vi "Auto Check Each Tube.vi"(0 "Ch 0 Leak":dbl, 1 "Cur Ch 0":refnum<vi>, 2 "Cur Ch 1":refnum<vi>, 5 "Tube #":i32, 7 "Ch 1 Leak":dbl, 9 "Barcodes in":string[](array[string]), 11 "BoardHandle in":T1, 12 "error in (no error)":errorcluster) -> (3 "Bool Bad Tubes":bool[](array[boolean]), 6 "Bad Tubes":string[](array[string]), 10 "error out":errorcluster, 13 "Channel 1 current":dbl, 14 "Channel 0 current":dbl, 15 "BoardHandle out":T1)   [LabVIEW 2020]
uses:
  Program Files/National Instruments/LabVIEW 2018/instr.lib/CAEN PSM/CAEN PSM.lvlib
panel:
  in  "User":string
  # "OUTPUTS"
  # "INPUTS"
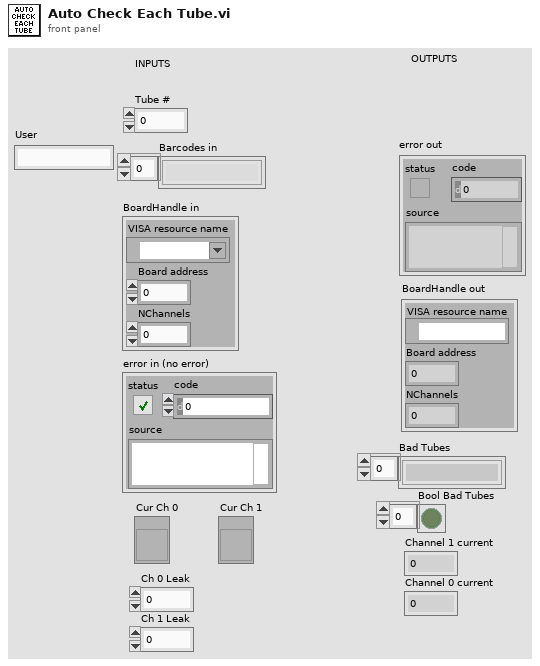
[diagram p1: front panel]
types:
  T1 = cluster{"VISA resource name":refnum<visa-resource-name>, "Board address":u8, "NChannels":u8}
  T2 = typedef "CAEN PSM.lvlib/BoardHandle.ctl" = cluster{"VISA resource name":refnum<visa-resource-name>, "Board address":u8, "NChannels":u8}
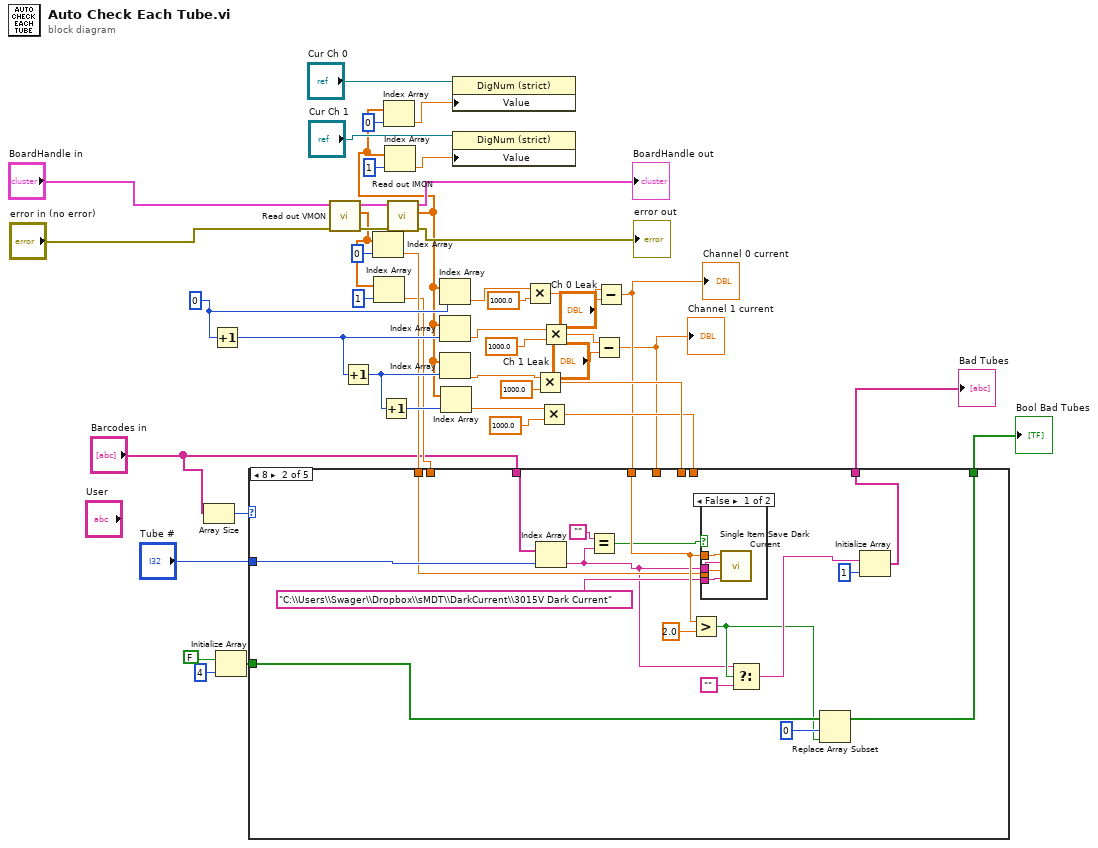
[diagram p0: block diagram]
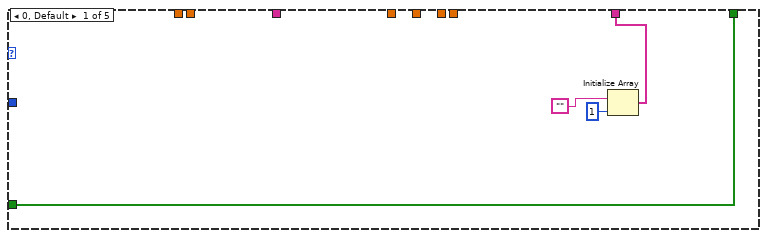
[diagram p2: hidden frame]
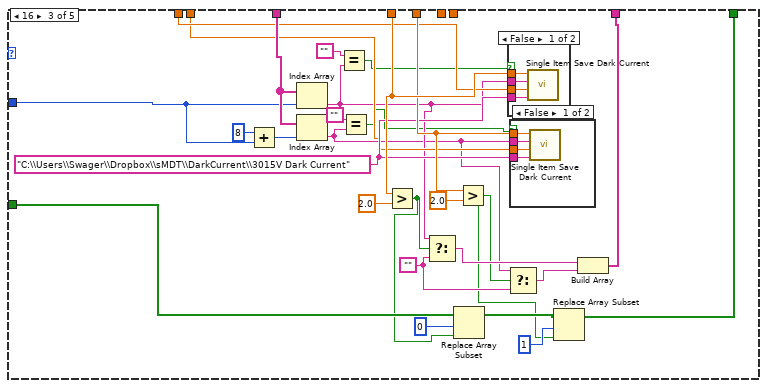
[diagram p4: hidden frame]
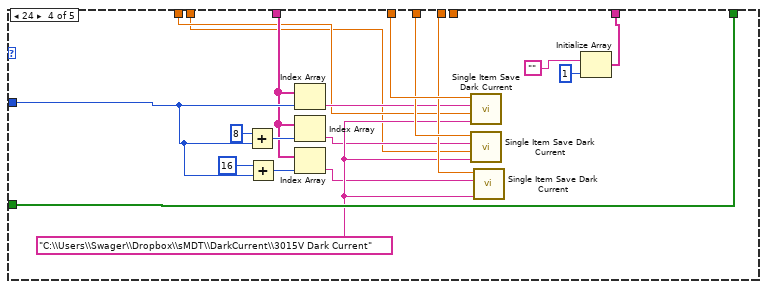
[diagram p7: hidden frame]
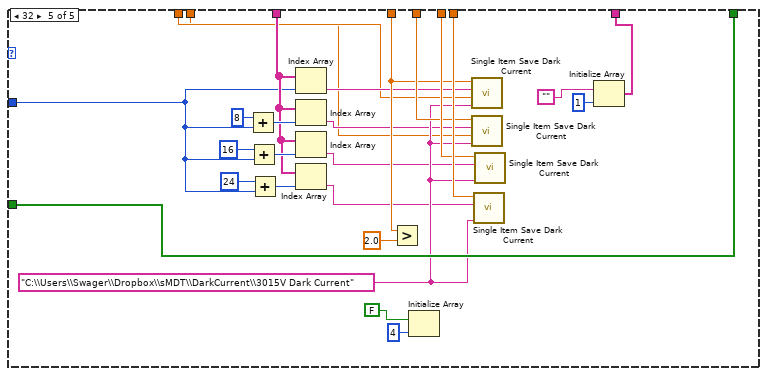
[diagram p8: hidden frame]
diagram:
  w35 = 0 ("index")
  n1 = Array Size(array="Barcodes in") -> (size(s)=w34:i32)
  n2 = Increment(x=w35) -> (x+1=w37:i32)
  n3 = Initialize Array(FALSE, 4 ("dimension size")) -> (w20:bool[])
  n4 = call "Read out VMON.vi"("error in (no error)"="error in (no error)", "BoardHandle"="BoardHandle in") -> ("error out"=w44:errorcluster, "VMon values (V)"=w4:dbl[], "BoardHandle out"=w43:T2)  [unwired: 7 in]
  n5 = Increment(x=w37) -> (x+1=w36:i32)
  n6 = Index Array(array=w4, index=0) -> (element=w3:dbl)
  n7 = Index Array(array=w4, index=1) -> (element=w2:dbl)
  n8 = Increment(x=w36) -> (x+1=w38:i32)
  n9 = call "Read out IMON.vi"("error in (no error)"=w44, "BoardHandle"=w43) -> ("error out"=→"error out":errorcluster, "IMon values (uA)"=w11:dbl[], "BoardHandle out"=→"BoardHandle out":T2)  [unwired: 6 in, 1 out]
  n10 = Index Array(array=w11, index=0) -> (element=w16:dbl)
  n11 = Index Array(array=w11, index=1) -> (element=w15:dbl)
  n12 = Index Array(array=w11, index=w35) -> (element=w45:dbl)
  n13 = Index Array(array=w11, index=w37) -> (element=w32:dbl)
  n14 = Index Array(array=w11, index=w36) -> (element=w29:dbl)
  n15 = Index Array(array=w11, index=w38) -> (element=w27:dbl)
  n16 = property class="DigNum (strict)"(reference="Cur Ch 0", "Value"=w16) -> ()  [unwired: 1 in, 2 out]
  n17 = property class="DigNum (strict)"(reference="Cur Ch 1", "Value"=w15) -> ()  [unwired: 1 in, 2 out]
  n18 = Multiply(x=w45, y=1000.0) -> (x*y=w23:dbl)
  n19 = Multiply(x=w29, y=1000.0) -> (x*y=w28:dbl)
  n20 = Multiply(x=w27, y=1000.0) -> (x*y=w25:dbl)
  n21 = Multiply(x=w32, y=1000.0) -> (x*y=w8:dbl)
  n22 = Subtract(x=w8, y="Ch 1 Leak") -> (x-y=w9:dbl)
  "Channel 1 current" <- w9
  n23 = Subtract(x=w23, y="Ch 0 Leak") -> (x-y=w12:dbl)
  "Channel 0 current" <- w12
  n24 = case shown="8" w34 {
    tunnel: w25 -> [_ _ _ _ w146]
    tunnel: w28 -> [_ _ _ w118 w145]
    tunnel: w9 -> [_ _ w81 w119 w144]
    tunnel: w12 -> [_ w60 w82 w120 w141]
    tunnel: "Barcodes in" -> [_ w67 w97 w121 w143]
    tunnel: "Tube #" -> [_ w66 w96 w122 w142]
    tunnel: [w48 w64 w91 w115 w135] -> w24
    tunnel: w20 -> [w47 w59 w88 w114 w134]
    tunnel: [w47 w56 w83 w114 w134] -> w19
    tunnel: w3 -> [_ w54 w79 w109 w128]
    tunnel: w2 -> [_ _ w78 w108 w127]
    frame 0, Default {
      n25 = Initialize Array("", 1 ("dimension size")) -> (w48:string[])
    }
    frame 8 {
      n26 = Index Array(array=w67, index=w66) -> (element=w53:string)
      n27 = Equal?(x="", y=w53) -> (x = y?=w51:bool)
      n28 = Greater?(x=w60, y=2.0) -> (0:w57:bool)
      n29 = case shown="False" w51 {
        tunnel: w60 -> [w71 _]
        tunnel: "C:\\Users\\Swager\\Dropbox\\sMDT\\DarkCurrent\\3015V Dark Current" ("Filename") -> [w70 _]
        tunnel: w54 -> [w69 _]
        tunnel: w53 -> [w68 _]
        frame False {
          n30 = call "Single Item Save Dark Current.vi"("Filename"=w70, "Voltage"=w69, "Barcode"=w68, "Current"=w71) -> ()  [unwired: 8 in]
        }
        frame True {
        }
      }
      n31 = Select(t=w53, s=w57, f="") -> (s? t:f=w61:string)
      n32 = Replace Array Subset(array=w59, new element=w57, index=0) -> (w56:bool[])
      n33 = Initialize Array(w61, 1 ("dimension size")) -> (w64:string[])
    }
    frame 16 {
      w80 = "C:\\Users\\Swager\\Dropbox\\sMDT\\DarkCurrent\\3015V Dark Current" ("Filename")
      w90 = ""
      n34 = Add(x=8, y=w96) -> (x+y=w99:i32)
      n35 = Index Array(array=w97, index=w96) -> (element=w77:string)
      n36 = Index Array(array=w97, index=w99) -> (element=w74:string)
      n37 = Equal?(x="", y=w77) -> (x = y?=w75:bool)
      n38 = Equal?(x="", y=w74) -> (x = y?=w72:bool)
      n39 = Greater?(x=w82, y=2.0) -> (0:w87:bool)
      n40 = Select(t=w77, s=w87, f=w90) -> (s? t:f=w93:string)
      n41 = Replace Array Subset(array=w88, new element=w87, index=0) -> (w85:bool[])
      n42 = Greater?(x=w81, y=2.0) -> (0:w84:bool)
      n43 = case shown="False" w75 {
        tunnel: w82 -> [w107 _]
        tunnel: w80 -> [w106 _]
        tunnel: w79 -> [w105 _]
        tunnel: w77 -> [w104 _]
        frame False {
          n44 = call "Single Item Save Dark Current.vi"("Filename"=w106, "Voltage"=w105, "Barcode"=w104, "Current"=w107) -> ()  [unwired: 8 in]
        }
        frame True {
        }
      }
      n45 = Select(t=w74, s=w84, f=w90) -> (s? t:f=w92:string)
      n46 = case shown="False" w72 {
        tunnel: w81 -> [w103 _]
        tunnel: w80 -> [w102 _]
        tunnel: w78 -> [w101 _]
        tunnel: w74 -> [w100 _]
        frame False {
          n47 = call "Single Item Save Dark Current.vi"("Filename"=w102, "Voltage"=w101, "Barcode"=w100, "Current"=w103) -> ()  [unwired: 8 in]
        }
        frame True {
        }
      }
      n48 = Replace Array Subset(array=w85, new element=w84, index=1) -> (w83:bool[])
      n49 = Build Array(w93, w92) -> (w91:string[])
    }
    frame 24 {
      w113 = "C:\\Users\\Swager\\Dropbox\\sMDT\\DarkCurrent\\3015V Dark Current" ("Filename")
      n50 = Add(x=8, y=w122) -> (x+y=w126:i32)
      n51 = Add(x=16, y=w122) -> (x+y=w124:i32)
      n52 = Index Array(array=w121, index=w122) -> (element=w112:string)
      n53 = Index Array(array=w121, index=w126) -> (element=w111:string)
      n54 = Index Array(array=w121, index=w124) -> (element=w110:string)
      n55 = call "Single Item Save Dark Current.vi"("Filename"=w113, "Voltage"=w109, "Barcode"=w112, "Current"=w120) -> ()  [unwired: 8 in]
      n56 = call "Single Item Save Dark Current.vi"("Filename"=w113, "Voltage"=w108, "Barcode"=w111, "Current"=w119) -> ()  [unwired: 8 in]
      n57 = call "Single Item Save Dark Current.vi"("Filename"=w113, "Barcode"=w110, "Current"=w118) -> ()  [unwired: 9 in]
      n58 = Initialize Array("", 1 ("dimension size")) -> (w115:string[])
    }
    frame 32 {
      w133 = "C:\\Users\\Swager\\Dropbox\\sMDT\\DarkCurrent\\3015V Dark Current" ("Filename")
      n59 = Add(x=8, y=w142) -> (x+y=w152:i32)
      n60 = Add(x=16, y=w142) -> (x+y=w150:i32)
      n61 = Add(x=24, y=w142) -> (x+y=w148:i32)
      n62 = Index Array(array=w143, index=w142) -> (element=w132:string)
      n63 = Index Array(array=w143, index=w152) -> (element=w131:string)
      n64 = Index Array(array=w143, index=w150) -> (element=w130:string)
      n65 = Index Array(array=w143, index=w148) -> (element=w129:string)
      n66 = Greater?(x=w141, y=2.0) -> ()  [unwired: 1 out]
      n67 = Initialize Array(FALSE, 4 ("dimension size")) -> ()  [unwired: 1 out]
      n68 = call "Single Item Save Dark Current.vi"("Filename"=w133, "Voltage"=w128, "Barcode"=w132, "Current"=w141) -> ()  [unwired: 8 in]
      n69 = call "Single Item Save Dark Current.vi"("Filename"=w133, "Voltage"=w127, "Barcode"=w131, "Current"=w144) -> ()  [unwired: 8 in]
      n70 = call "Single Item Save Dark Current.vi"("Filename"=w133, "Barcode"=w129, "Current"=w146) -> ()  [unwired: 9 in]
      n71 = call "Single Item Save Dark Current.vi"("Filename"=w133, "Barcode"=w130, "Current"=w145) -> ()  [unwired: 9 in]
      n72 = Initialize Array("", 1 ("dimension size")) -> (w135:string[])
    }
  }
  "Bad Tubes" <- w24
  "Bool Bad Tubes" <- w19
